vi "getWfFromShwfsFile.vi"(8 "error in (no error)":errorcluster, 10 "Wfs Err Data":path=path "/home/ttsai/Documents/stash/ts_tcs_ofc/testData/shwfs_wfs_error.txt", 11 "ZTAAC in":refnum<class "ZTAAC.lvclass">) -> (0 "error out":errorcluster, 1 "Sensor Name":string[](array[string])=["R:4,4 S:0,0", "R:0,4 S:2,0", "R:0,0 S:2,2", "R:4,0 S:0,2"], 2 "Wavefront Error":dbl[][](array[numeric]), 3 "ZTAAC out":refnum<class "ZTAAC.lvclass">)   [LabVIEW 2016, in "OfcFunc.lvlib" / "ZTAAC.lvclass"]
doc: "Get the wavefront error from the SHWFS file."
uses:
  ZTAAC.lvclass
  ZTAAC.lvclass/ZTAAC.ctl
  OptStateEsti/OptStateEsti.lvclass
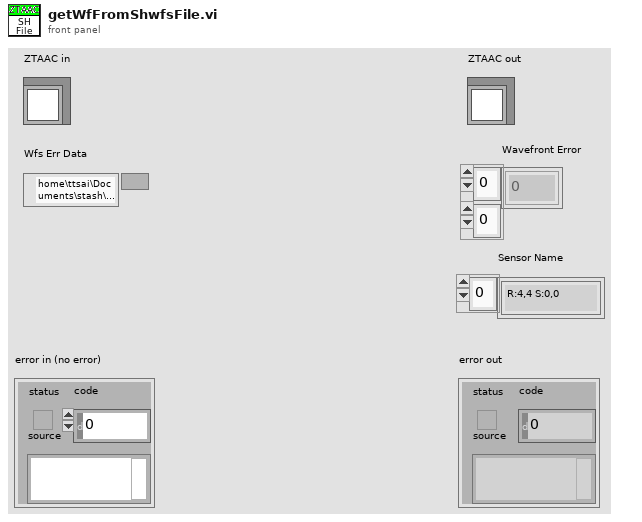
[diagram p1: front panel]
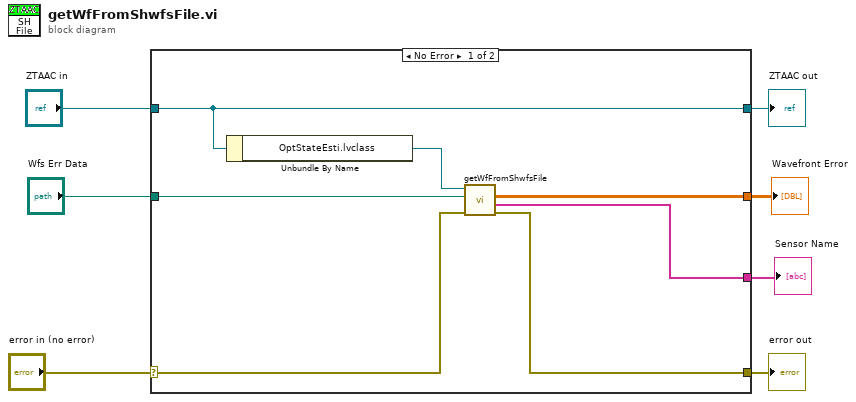
[diagram p0: block diagram]
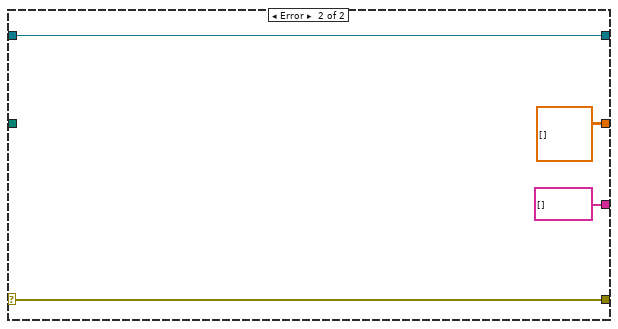
[diagram p2: hidden frame]
diagram:
  n1 = case shown="No Error" "error in (no error)" {
    selector: "error in (no error)" -> [w11 w18]
    tunnel: [w10 w18] -> w6
    tunnel: [w14 w17] -> w4
    tunnel: "ZTAAC in" -> [w14 w17]
    tunnel: "Wfs Err Data" -> [w12 _]
    tunnel: [w9 dbl[][] [] ("Wavefront Error")] -> w2
    tunnel: [w8 string[] [] ("Sensor Name")] -> w1
    frame No Error {
      n2 = Unbundle By Name(w14) -> ("OptStateEsti.lvclass"=w13:refnum<class "OptStateEsti.lvclass">)
      n3 = call "getWfFromShwfsFile.vi"("error in (no error)"=w11, "Wfs Err Data"=w12, "OptStateEsti in"=w13) -> ("error out"=w10:errorcluster, "Sensor Name"=w8:string[], "Wavefront Error"=w9:dbl[][])  [unwired: 5 in, 1 out]
    }
    frame Error {
    }
  }
  "error out" <- w6
  "ZTAAC out" <- w4
  "Sensor Name" <- w1
  "Wavefront Error" <- w2
